vi "TagQueryCurrentIntValuesRequest_Parse.vi"(8 "error in (no error)":errorcluster, 11 "Message":T5) -> (0 "error out":errorcluster, 1 "Body":T1, 2 "Header":T3, 3 "TagQueryCurrentIntValuesRequest":T2)   [LabVIEW 2017]
uses:
  <vilib>/addons/InsightCM/MessageBus/Base/controls/Message.ctl
  <vilib>/addons/InsightCM/MessageBus/Base/controls/MessageHeader.ctl
  <vilib>/addons/InsightCM/MessageBus/Base/controls/KeyValuePair.ctl
  <vilib>/addons/InsightCM/MessageBus/MessageLibrary/Tag/controls/TagQueryCurrentIntValuesRequest.ctl
  <vilib>/addons/InsightCM/MessageBus/MessageLibrary/Tag/controls/TagQueryCurrentIntValuesRequestBody.ctl
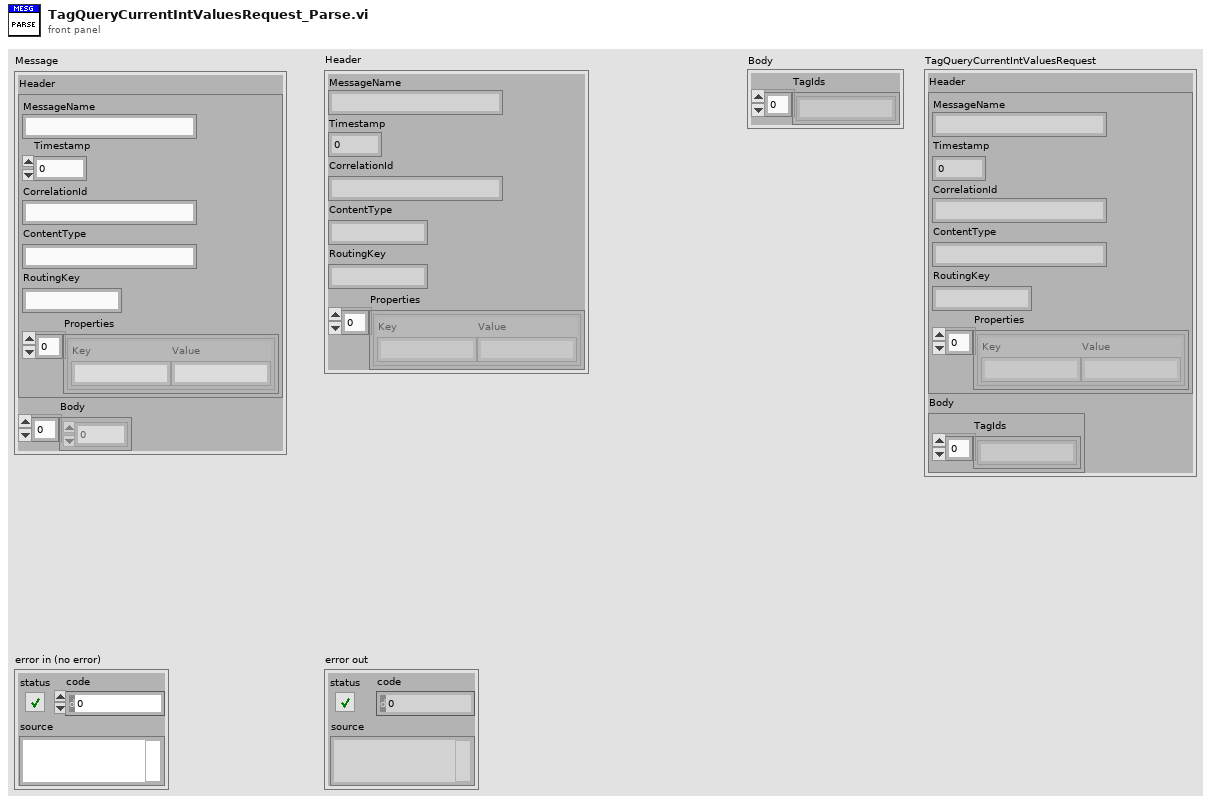
[diagram p1: front panel]
types:
  T1 = typedef "TagQueryCurrentIntValuesRequestBody.ctl" = cluster{"TagIds":string[]}
  T2 = typedef "TagQueryCurrentIntValuesRequest.ctl" = cluster{"Header":T3, "Body":T1}
  T3 = typedef "MessageHeader.ctl" = cluster{"MessageName":string, "Timestamp":i64, "CorrelationId":string, "ContentType":string, "RoutingKey":string, "Properties":T4[]}
  T4 = typedef "KeyValuePair.ctl" = cluster{"Key":string, "Value":string}
  T5 = typedef "Message.ctl" = cluster{"Header":T3, "Body":u8[]}
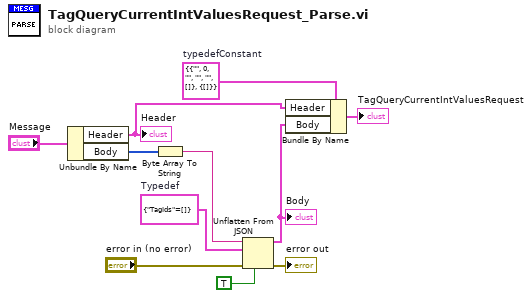
[diagram p0: block diagram]
diagram:
  w3 = T2 {"Header"={"MessageName"="", "Timestamp"=0, "CorrelationId"="", "ContentType"="", "RoutingKey"="", "Properties"=[]}, "Body"={"TagIds"=[]}}  # typedefConstant
  w7 = T1 {"TagIds"=[]}  # Typedef
  n1 = Unbundle By Name("Message") -> ("Header"=w9:T3, "Body"=w1:u8[])
  "Header" <- w9
  n2 = Byte Array To String(unsigned byte array=w1) -> (string=w6:string)
  n3 = Unflatten From JSON(JSON string=w6, type and defaults=w7, default null elements? (F)=TRUE, error in (no error)="error in (no error)") -> (value=w5:T1, error out=→"error out":errorcluster)  [unwired: 3 in]
  "Body" <- w5
  n4 = Bundle By Name(cluster=w3, "Header"=w9, "Body"=w5) -> (→"TagQueryCurrentIntValuesRequest":T2)
